vi "03Foot.vi"() -> ()   [LabVIEW 2015]
uses:
  <vilib>/DAQmx/read.llb/DAQmx Read (Digital 1D U8 1Chan NSamp).vi
  <vilib>/Instr/_visa.llb/VISA Configure Serial Port (Serial Instr).vi
  <vilib>/DAQmx/create/channels.llb/DAQmx Create Channel (DI-Digital Input).vi
  <vilib>/DAQmx/configure/timing.llb/DAQmx Timing (Sample Clock).vi
  <vilib>/DAQmx/miscellaneous.llb/DAQmx Fill In Error Info.vi
  <vilib>/Utility/file.llb/Write Delimited Spreadsheet (I64).vi
panel:
  out "MPH READ":u8
  out "appended path":path
  out "Waveform Graph":dbl[](graph)
  out "String":string
  out "x-y":u32
  out "stopping":bool
  in  "lines":tag="DAQMod1/port0"
  in  "Serial Port":refnum<visa-resource-name>="COM8"
  in  "stop":bool
  out "MPH":dbl min=0.0 max=12.0 step=0.1 format="%.1f"
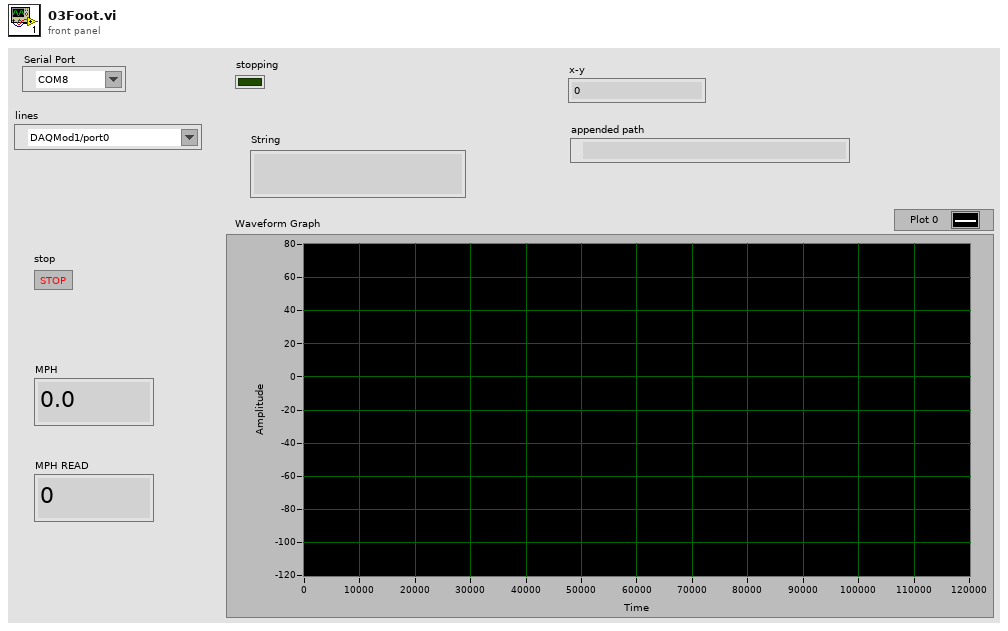
[diagram p1: front panel]
types:
  T1 = enum16{"Initialize", "SetMPH", "GetData", "CheckTiming", "CompressWave", "StartDAQ", "StopDAQ"}
  T2 = enum16{"Initialize", "SetMPH", "GetData", "CheckTiming"}
  T3 = enum16{"Initialize", "SetMPH", "GetData", "CheckTiming", "CompressWave", "StartDAQ"}
  T4 = enum16{"Initialize", "SetMPH", "GetData", "CheckTiming", "CompressWave"}
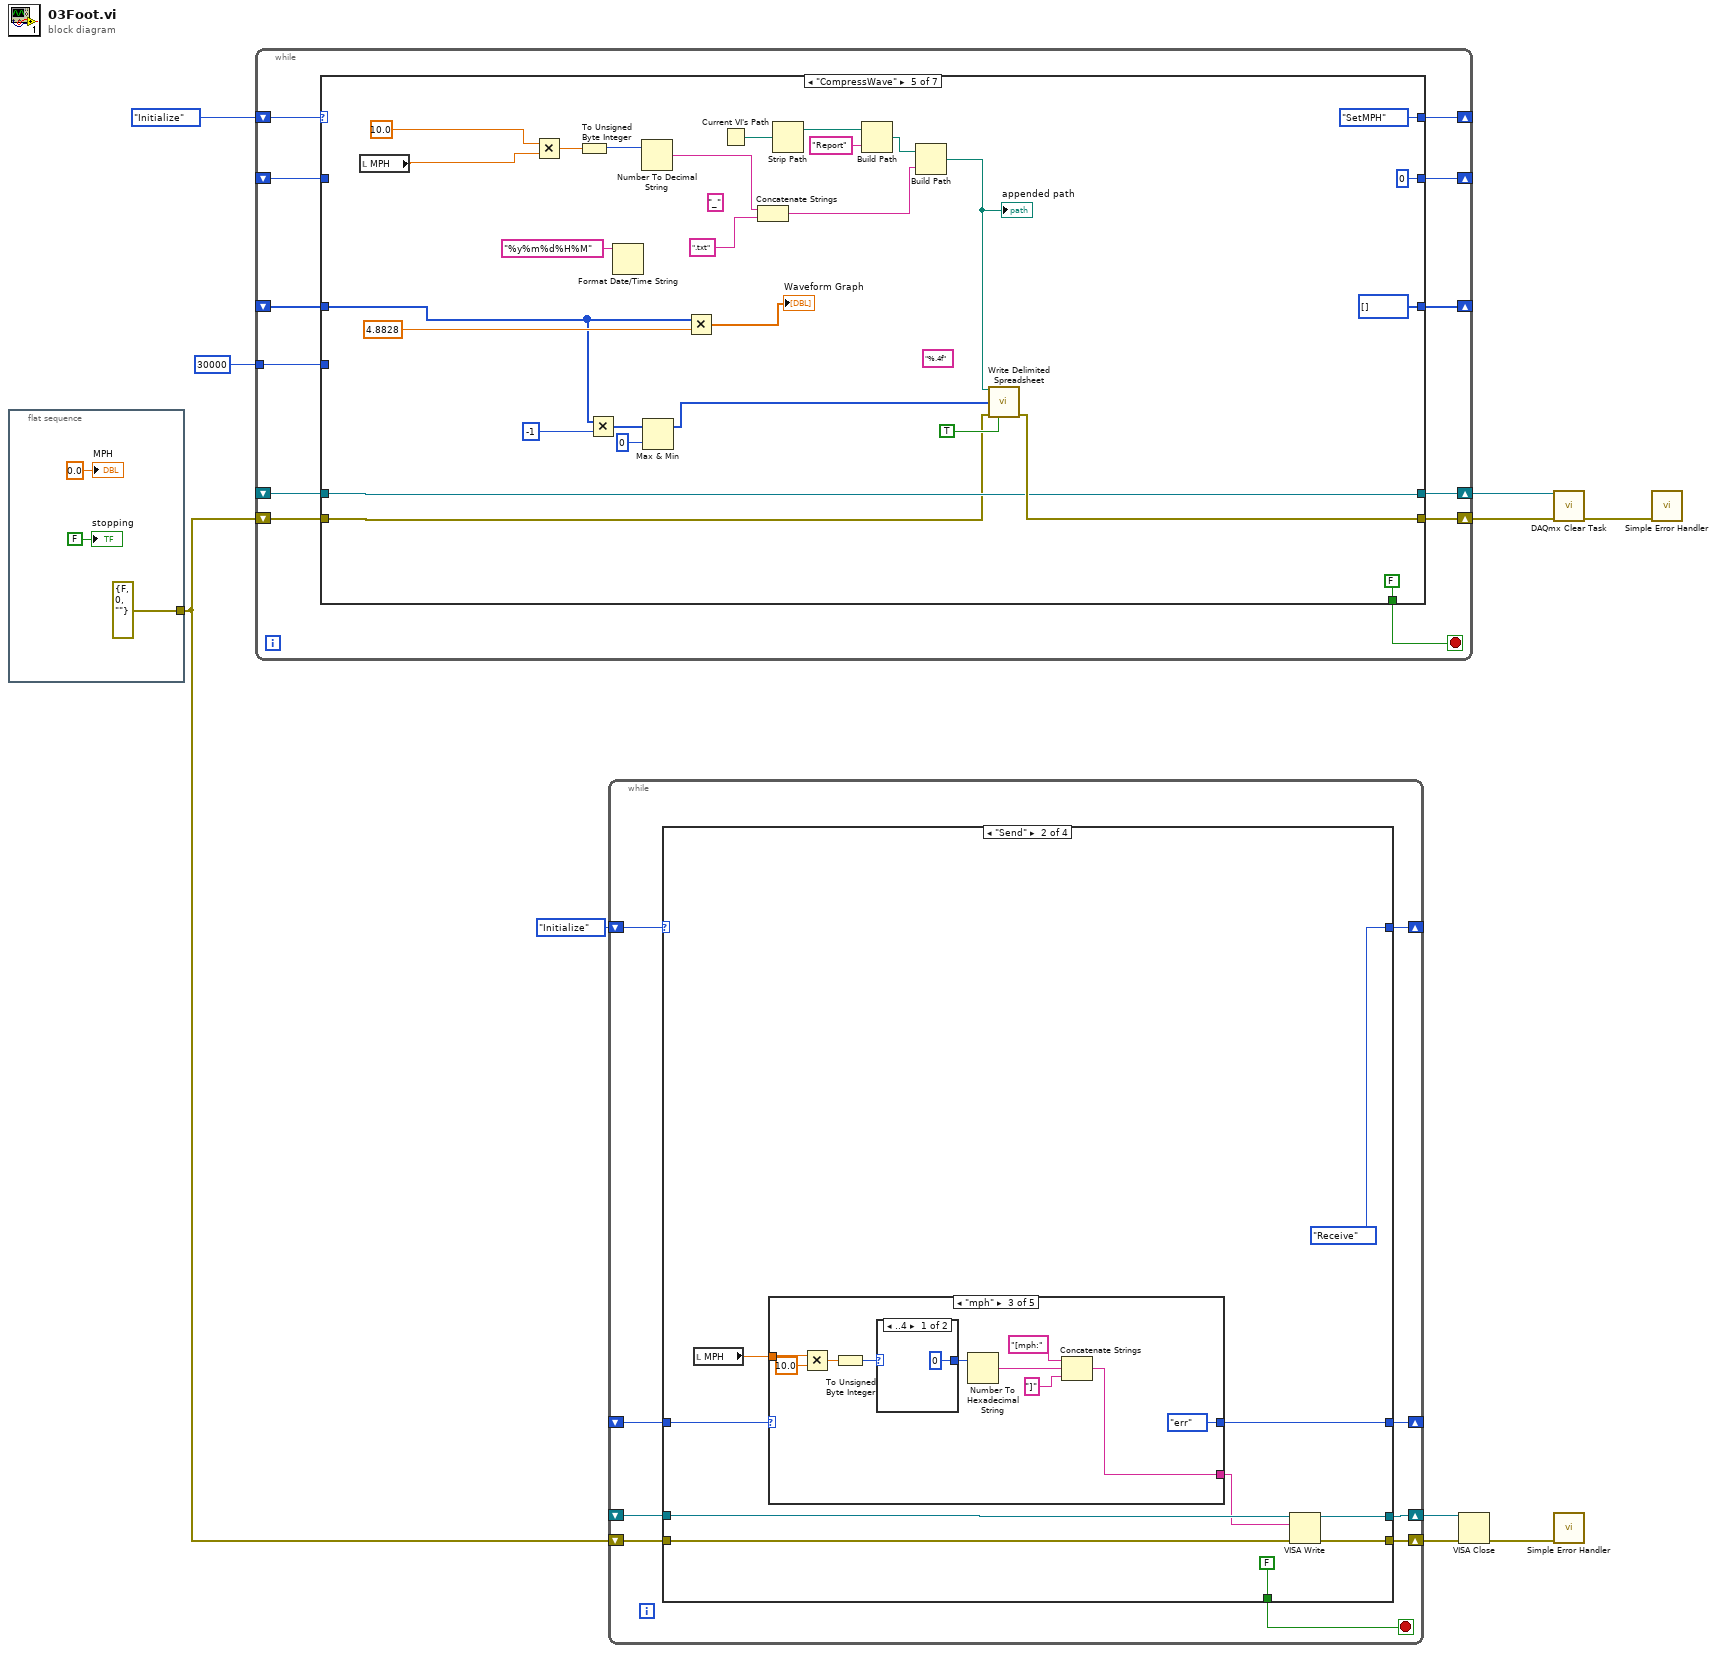
[diagram p0: block diagram]
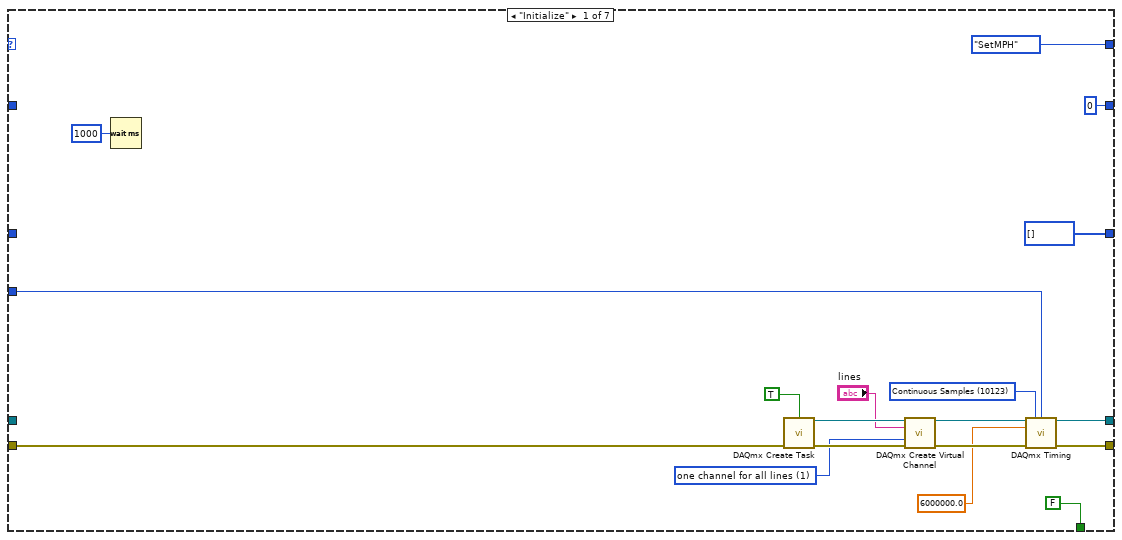
[diagram p2: hidden frame]
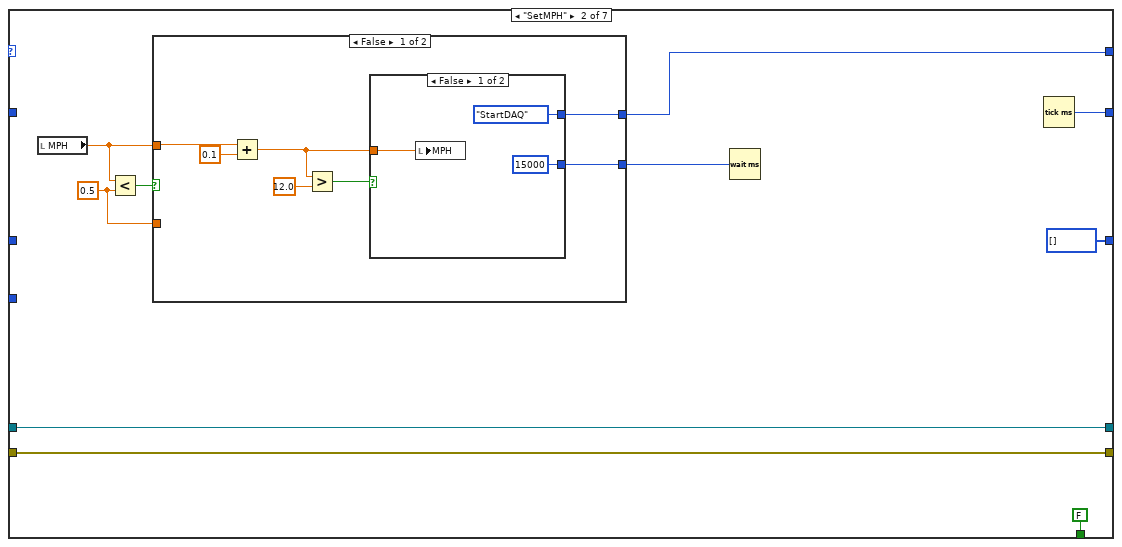
[diagram p3: hidden frame]
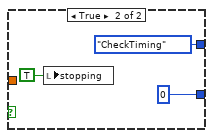
[diagram p4: hidden frame]
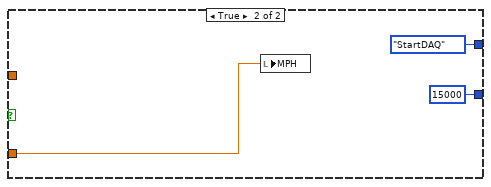
[diagram p5: hidden frame]
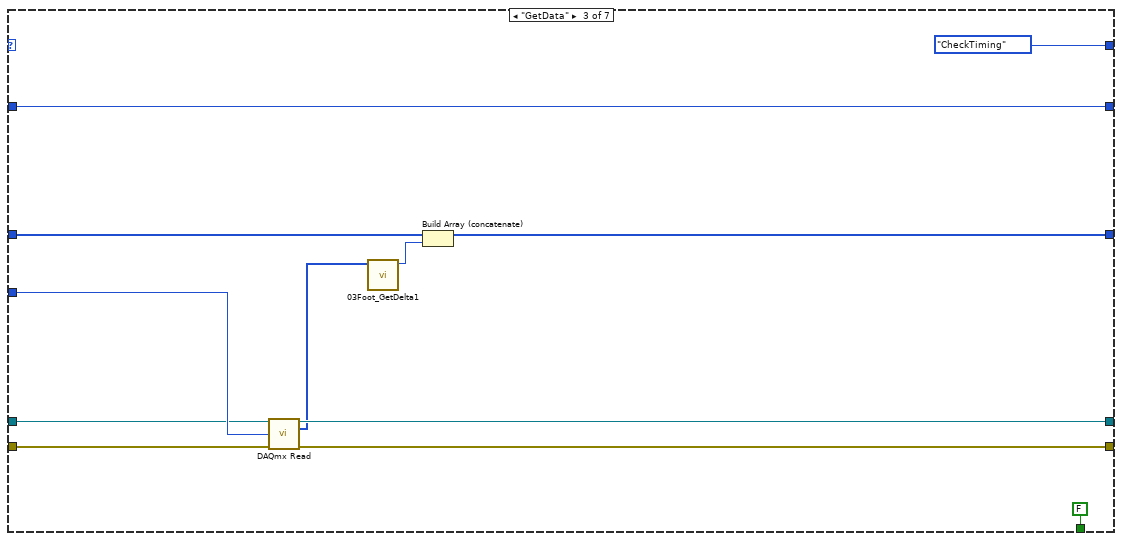
[diagram p6: hidden frame]
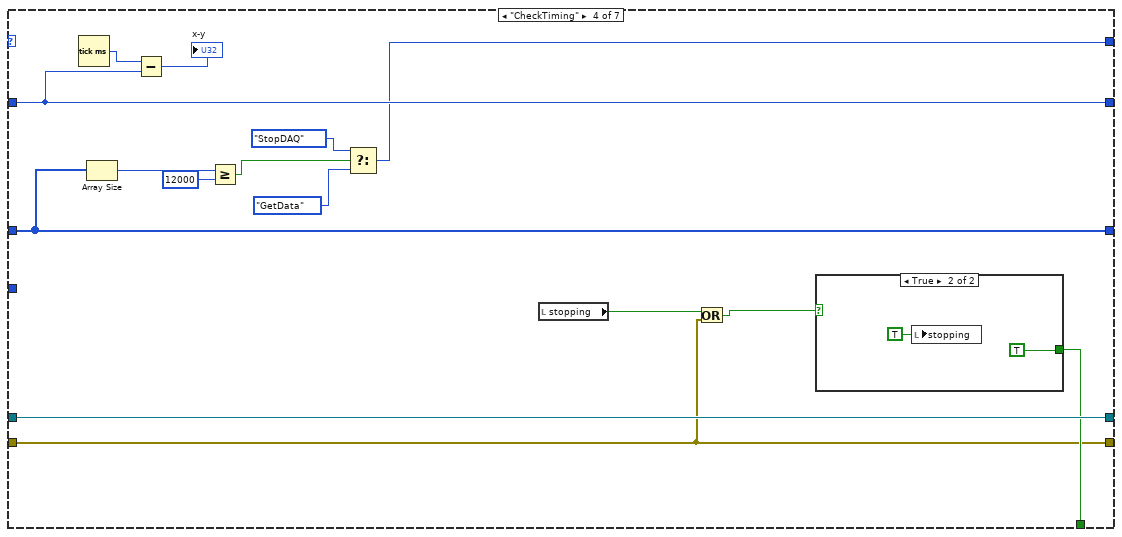
[diagram p7: hidden frame]
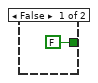
[diagram p8: hidden frame]
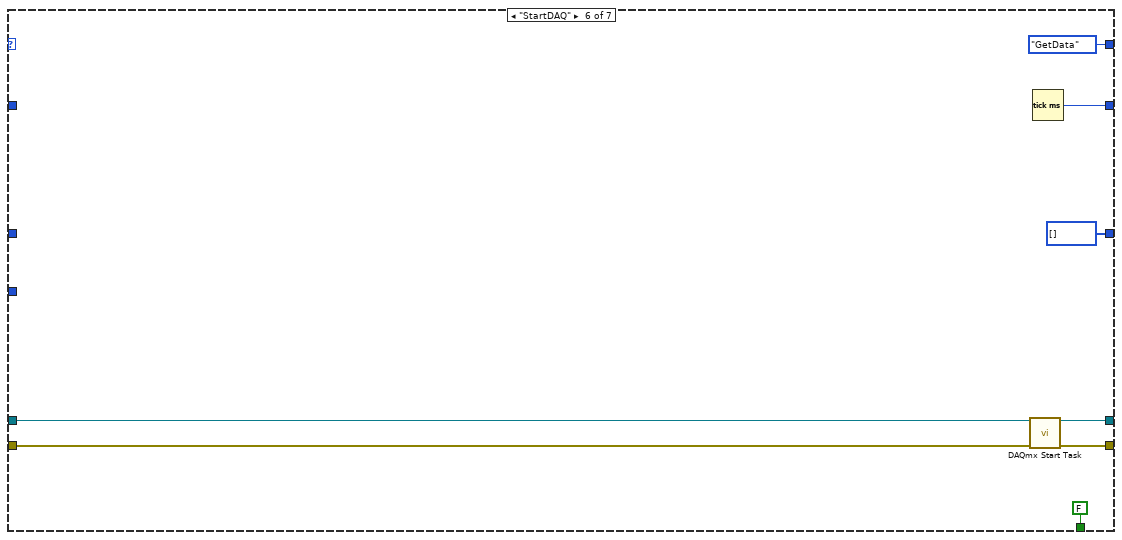
[diagram p9: hidden frame]
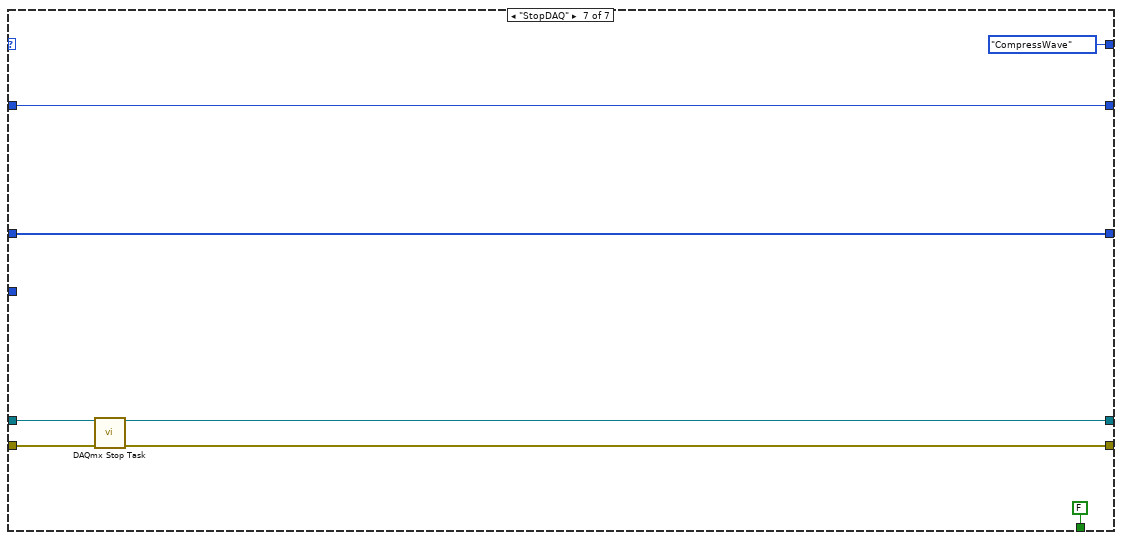
[diagram p10: hidden frame]
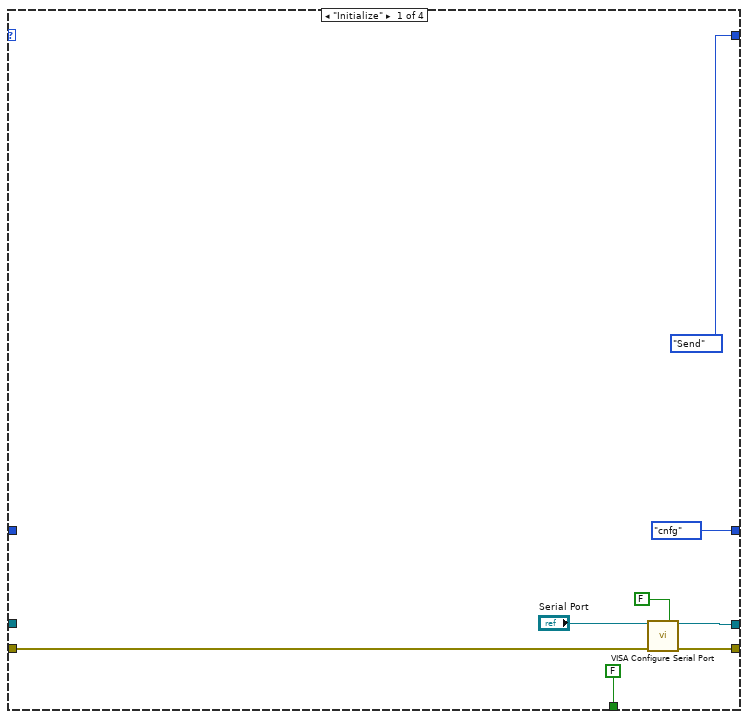
[diagram p11: hidden frame]
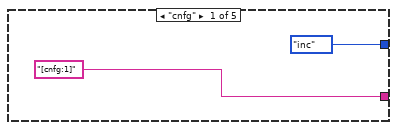
[diagram p12: hidden frame]
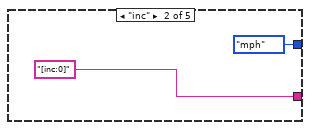
[diagram p13: hidden frame]
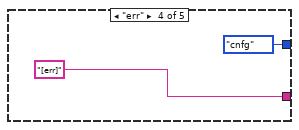
[diagram p15: hidden frame]
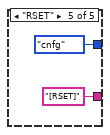
[diagram p16: hidden frame]
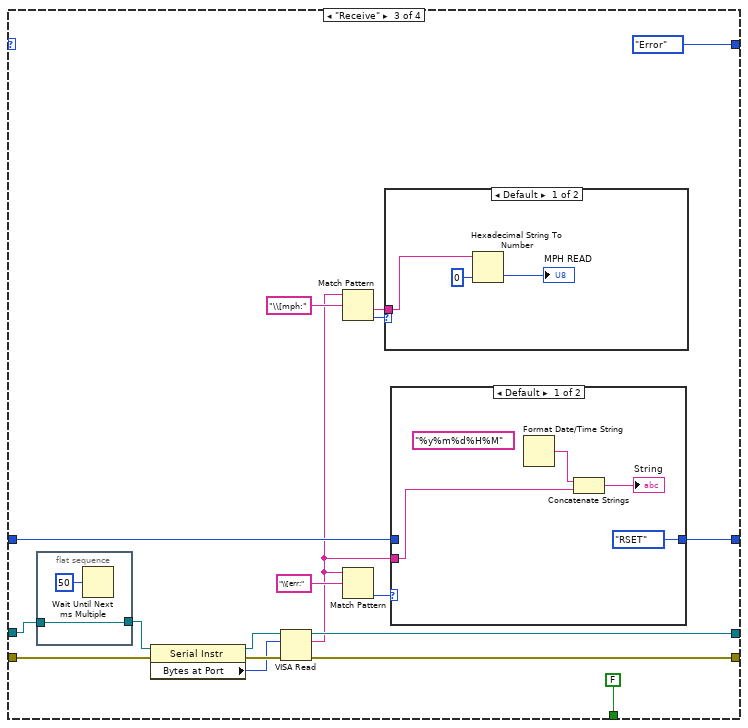
[diagram p17: hidden frame]
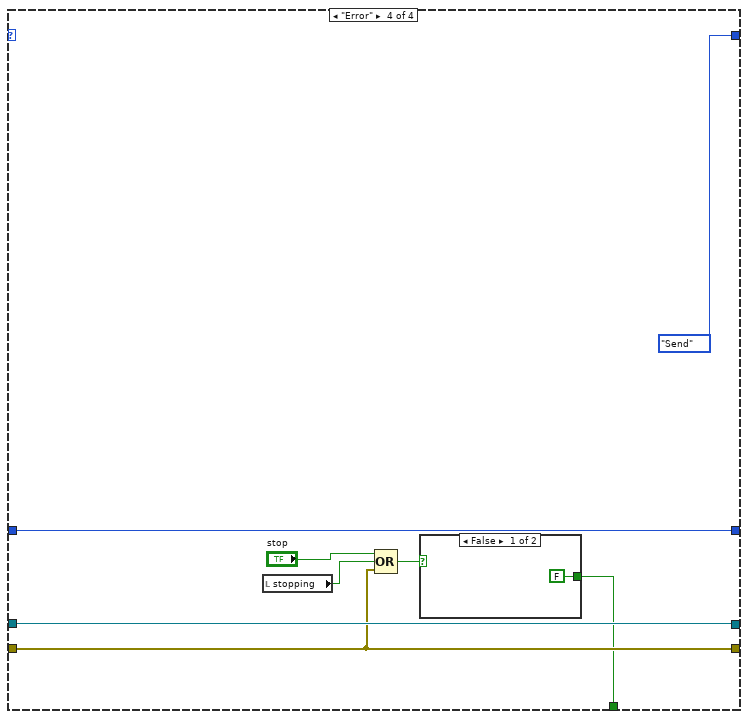
[diagram p20: hidden frame]
diagram:
  n1 = flat-sequence {
    tunnel: [errorcluster {"status"=FALSE, "code"=0, "source"=""} ("error constant")] -> w2
    frame #0 {
      "stopping" <- FALSE ("stopping")
      "MPH" <- 0.0 ("MPH")
    }
  }
  n2 = while {
    shift-right: [w24] -> _
    shift-left: T1."Initialize" -> [w25]
    shift-right: [w22] -> w4
    shift-left: _ -> [w20]
    shift-right: [w21] -> w5
    shift-left: w2 -> [w19]
    shift-right: [w18] -> _
    shift-left: _ -> [w17]
    tunnel: 30000 ("samples per channel") -> [w16]
    shift-right: [w15] -> _
    shift-left: _ -> [w14]
    stop <- w23 stop-if-true
    n3 = case shown="\"CompressWave\"" w25 {
      tunnel: [T2."SetMPH" w44 T4."CheckTiming" w86 T4."SetMPH" T3."GetData" T1."CompressWave"] -> w24
      tunnel: [FALSE FALSE FALSE w92 FALSE FALSE FALSE] -> w23
      tunnel: [w31 w47 w77 w96 w101 w130 w139] -> w22
      tunnel: [w30 w46 w78 w88 w123 w131 w138] -> w21
      tunnel: w20 -> [_ w47 w71 w96 w101 w129 w141]
      tunnel: w19 -> [w26 w46 w70 w88 w100 w128 w140]
      tunnel: [u32 0 w45 w80 w91 u32 0 w134 w136] -> w18
      tunnel: w17 -> [_ _ w80 w91 _ _ w136]
      tunnel: w16 -> [w29 _ w79 _ _ _ _]
      tunnel: [i32[] [] i32[] [] w76 w85 i32[] [] i32[] [] w142] -> w15
      tunnel: w14 -> [_ _ w75 w85 w107 _ w142]
      frame "Initialize" {
        w28 = 10123 items=["Finite Samples"=10178, "Continuous Samples"=10123, "Hardware Timed Single Point"=12522] ("sample mode")
        w41 = 1 items=["one channel for each line", "one channel for all lines"] ("line grouping")
        n4 = Wait (ms)(milliseconds to wait=u32 1000) -> ()  [unwired: 1 out]
        n5 = call <vilib>:"DAQmx Create Task.vi"("auto cleanup"=TRUE, "error in"=w26) -> ("task out"=w43:refnum<k21>, "error out"=w42:errorcluster)  [unwired: 12 in]
        n6 = call-poly <vilib>:"DAQmx Create Virtual Channel.vi"("task in"=w43, "lines"="lines", "line grouping"=w41, "error in"=w42) -> ("task out"=w32:refnum<k21>, "error out"=w33:errorcluster)  [unwired: 10 in]
        n7 = call-poly <vilib>:"DAQmx Timing.vi"("task/channels in"=w32, "sample mode"=w28, "samples per channel"=w29, "rate"=6000000.0, "error in"=w33) -> ("task out"=w31:refnum<k21>, "error out"=w30:errorcluster)  [unwired: 9 in]
      }
      frame "SetMPH" {
        w48 = 0.5 ("y")
        n8 = local read "MPH"() -> (w51:dbl)
        n9 = Less?(x=w51, y=w48) -> (x < y?=w52:bool)
        n10 = case shown="False" w52 {
          tunnel: w51 -> [w56 _]
          tunnel: [w58 u32 15000 ("milliseconds to wait")] -> w50
          tunnel: w48 -> [_ w68]
          tunnel: [w54 T3."StartDAQ"] -> w44
          frame False {
            n11 = Add(x=w56, y=0.1) -> (x+y=w55:dbl)
            n12 = Greater?(x=w55, y=12.0) -> (0:w59:bool)
            n13 = case shown="False" w59 {
              tunnel: w55 -> [w62 _]
              tunnel: [u32 15000 ("milliseconds to wait") u32 0 ("milliseconds to wait")] -> w58
              tunnel: [T3."StartDAQ" T3."CheckTiming"] -> w54
              frame False {
                n14 = local write "MPH"(w62) -> ()
              }
              frame True {
                n15 = local write "stopping"(TRUE ("stopping")) -> ()
              }
            }
          }
          frame True {
            n16 = local write "MPH"(w68) -> ()
          }
        }
        n17 = Wait (ms)(milliseconds to wait=w50) -> ()  [unwired: 1 out]
        n18 = Tick Count (ms)() -> (millisecond timer value=w45:u32)
      }
      frame "GetData" {
        n19 = call-poly <vilib>:"DAQmx Read.vi"("task/channels in"=w71, "number of samples per channel"=w79, "error in"=w70) -> ("task out"=w77:refnum<k21>, "data"=w72:u8[], "error out"=w78:errorcluster)  [unwired: 10 in]
        n20 = call "03Foot_GetDelta1.vi"("Array"=w72) -> ("Wave1 Data"=w73:i32)  [unwired: 10 in]
        n21 = Build Array (concatenate)(w75, w73) -> (w76:i32[])
      }
      frame "CheckTiming" {
        n22 = Tick Count (ms)() -> (millisecond timer value=w95:u32)
        n23 = Array Size(array=w85) -> (size(s)=w84:i32)
        n24 = Subtract(x=w95, y=w91) -> (x-y=→"x-y":u32)
        n25 = Greater Or Equal?(x=w84, y=12000) -> (x >= y?=w87:bool)
        n26 = Select(t=T1."StopDAQ", s=w87, f=T1."GetData") -> (s? t:f=w86:T1)
        n27 = local read "stopping"() -> (w90:bool)
        n28 = Or(x=w90, y=w88) -> (x .or. y?=w89:bool)
        n29 = case shown="True" w89 {
          tunnel: [FALSE TRUE] -> w92
          frame False {
          }
          frame True {
            n30 = local write "stopping"(TRUE ("stopping")) -> ()
          }
        }
      }
      frame "CompressWave" {
        (unwired) "%.4f" ("format (%.3f)")
        (unwired) "_" ("string")
        n31 = local read "MPH"() -> (w106:dbl)
        n32 = Multiply(x=10.0, y=w106) -> (x*y=w112:dbl)
        n33 = To Unsigned Byte Integer(number=w112) -> (unsigned 8bit integer=w111:u8)
        n34 = Multiply(x=w107, y=-1) -> (x*y=w104:i32[])
        n35 = Format Date/Time String(time format string (%c)="%y%m%d%H%M") -> ()  [unwired: 2 in, 1 out]
        n36 = Number To Decimal String(number=w111) -> (decimal integer string=w110:string)  [unwired: 1 in]
        n37 = Max & Min(x=w104, y=0) -> (max(x,y)=w102:i32[])  [unwired: 1 out]
        n38 = Multiply(x=w107, y=4.8828) -> (x*y=→"Waveform Graph":dbl[])
        n39 = Current VI's Path() -> (path=w121:path)
        n40 = Concatenate Strings(w110, ".txt" ("string")) -> (w115:string)
        n41 = Strip Path(path=w121) -> (stripped path=w118:path)  [unwired: 1 out]
        n42 = Build Path(base path=w118, name or relative path="Report") -> (appended path=w116:path)
        n43 = Build Path(base path=w116, name or relative path=w115) -> (appended path=w114:path)
        "appended path" <- w114
        n44 = call-poly <vilib>:"Write Delimited Spreadsheet.vi"("file path (dialog if empty)"=w114, "1D data"=w102, "error in (no error)"=w100, "transpose? (F)"=TRUE) -> ("error out"=w123:errorcluster)  [unwired: 10 in, 1 out]
      }
      frame "StartDAQ" {
        n45 = call <vilib>:"DAQmx Start Task.vi"("task/channels in"=w129, "error in"=w128) -> ("task out"=w130:refnum<k21>, "error out"=w131:errorcluster)  [unwired: 12 in]
        n46 = Tick Count (ms)() -> (millisecond timer value=w134:u32)
      }
      frame "StopDAQ" {
        n47 = call <vilib>:"DAQmx Stop Task.vi"("task/channels in"=w141, "error in"=w140) -> ("task out"=w139:refnum<k21>, "error out"=w138:errorcluster)  [unwired: 12 in]
      }
    }
  }
  n48 = while {
    shift-right: [w148] -> w8
    shift-left: w2 -> [w152]
    shift-right: [w149] -> w9
    shift-left: _ -> [w151]
    shift-right: [w147] -> _
    shift-left: enum16{"Initialize", "Send", "Receive", "Error"}."Initialize" -> [w150]
    shift-right: [w146] -> _
    shift-left: _ -> [w145]
    stop <- w144 stop-if-true
    n49 = case shown="\"Send\"" w150 {
      tunnel: w152 -> [w156 w168 w204 w220]
      tunnel: w151 -> [_ w167 w203 w224]
      tunnel: [w158 w170 w202 w224] -> w149
      tunnel: [w157 w169 w195 w220] -> w148
      tunnel: [enum16{"Initialize", "Send", "Receive", "Error"}."Send" enum16{"Initialize", "Send", "Receive", "Error"}."Receive" enum16{"Initialize", "Send", "Receive", "Error"}."Error" enum16{"Initialize", "Send", "Receive", "Error"}."Send"] -> w147
      tunnel: [enum16{"cnfg", "inc", "mph", "err", "RSET"}."cnfg" w164 w197 w225] -> w146
      tunnel: w145 -> [_ w165 w196 w225]
      tunnel: [FALSE FALSE FALSE w219] -> w144
      frame "Initialize" {
        n50 = call-poly "VISA Configure Serial Port"("VISA resource name"="Serial Port", "Enable Termination\nChar (T)"=FALSE ("Enable Termination\nChar (T)"), "error in (no error)"=w156) -> ("VISA resource name out"=w158:refnum<visa-resource-name>, "error out"=w157:errorcluster)  [unwired: 11 in]
      }
      frame "Send" {
        n51 = local read "MPH"() -> (w161:dbl)
        n52 = case shown="\"mph\"" w165 {
          tunnel: ["[cnfg:1]" "[inc:0]" w175 "[err]" "[RSET]"] -> w166
          tunnel: w161 -> [_ _ w184 _ _]
          tunnel: [enum16{"cnfg", "inc", "mph", "err", "RSET"}."inc" enum16{"cnfg", "inc", "mph", "err", "RSET"}."mph" enum16{"cnfg", "inc", "mph", "err", "RSET"}."err" enum16{"cnfg", "inc", "mph", "err", "RSET"}."cnfg" enum16{"cnfg", "inc", "mph", "err", "RSET"}."cnfg"] -> w164
          frame "cnfg" {
          }
          frame "inc" {
          }
          frame "mph" {
            n53 = Multiply(x=w184, y=10.0) -> (x*y=w178:dbl)
            n54 = To Unsigned Byte Integer(number=w178) -> (unsigned 8bit integer=w177:u8)
            n55 = case shown="..4" w177 {
              selector: w177 -> [_ w186]
              tunnel: [u8 0 w186] -> w176
              frame ..4 {
              }
              frame 5.. {
              }
            }
            n56 = Number To Hexadecimal String(2:w176) -> (0:w181:string)  [unwired: 1 in]
            n57 = Concatenate Strings("[mph:" ("string"), w181, "]" ("string")) -> (w175:string)
          }
          frame "err" {
          }
          frame "RSET" {
          }
        }
        n58 = VISA Write(VISA resource name=w167, write buffer=w166, error in (no error)=w168) -> (VISA resource name out=w170:refnum<visa-resource-name>, error out=w169:errorcluster)  [unwired: 1 out]
      }
      frame "Receive" {
        n59 = flat-sequence {
          tunnel: w203 -> [w217]
          tunnel: [w217] -> w208
          frame #0 {
            n60 = Wait Until Next ms Multiple(millisecond multiple=u32 50) -> ()  [unwired: 1 out]
          }
        }
        n61 = property class="Serial Instr"(reference=w208, error in=w204) -> (reference out=w206:refnum<visa-resource-name>, error out=w207:errorcluster, "Bytes at Port"=w205:u32)
        n62 = VISA Read(VISA resource name=w206, byte count=w205, error in (no error)=w207) -> (VISA resource name out=w202:refnum<visa-resource-name>, read buffer=w193:string, error out=w195:errorcluster)  [unwired: 1 out]
        n63 = Match Pattern(string=w193, regular expression="\\[mph:") -> (after substring=w191:string, offset past match=w192:i32)  [unwired: 1 in, 2 out]
        n64 = Match Pattern(string=w193, regular expression="\\[err:") -> (offset past match=w198:i32)  [unwired: 1 in, 3 out]
        n65 = case shown="Default" w192 {
          tunnel: w191 -> [w211 _]
          frame Default {
            n66 = Hexadecimal String To Number(string=w211, default (0uL)=u8 0 ("default (0 I32)")) -> (number=→"MPH READ":u8)  [unwired: 1 in, 1 out]
          }
          frame -1 {
          }
        }
        n67 = case shown="Default" w198 {
          tunnel: [enum16{"cnfg", "inc", "mph", "err", "RSET"}."RSET" w216] -> w197
          tunnel: w196 -> [_ w216]
          tunnel: w193 -> [w212 _]
          frame Default {
            (unwired) "%y%m%d%H%M" ("time format string (%c)")
            n68 = Format Date/Time String() -> (date/time string=w213:string)  [unwired: 3 in]
            n69 = Concatenate Strings(w213, w212) -> (→"String":string)
          }
          frame -1 {
          }
        }
      }
      frame "Error" {
        n70 = local read "stopping"() -> (w221:bool)
        n71 = Compound Arithmetic op=OR("stop", w221, w220) -> (w223:bool)
        n72 = case shown="False" w223 {
          tunnel: [FALSE TRUE] -> w219
          frame False {
          }
          frame True {
            n73 = local write "stopping"(TRUE ("stopping")) -> ()
          }
        }
      }
    }
  }
  n74 = VISA Close(VISA resource name=w9, error in (no error)=w8) -> (error out=w7:errorcluster)
  n75 = call <vilib>:"DAQmx Clear Task.vi"("task in"=w4, "error in"=w5) -> ("error out"=w3:errorcluster)  [unwired: 13 in]
  n76 = call <vilib>:"Simple Error Handler.vi"("error in (no error)"=w7) -> ()  [unwired: 4 in, 5 out]
  n77 = call <vilib>:"Simple Error Handler.vi"("error in (no error)"=w3) -> ()  [unwired: 4 in, 5 out]
